vi "hamamatsuReadIndexesOnly.vi"   [LabVIEW 2017]
uses:
  globalDevices.vi
  globalUtilities.vi
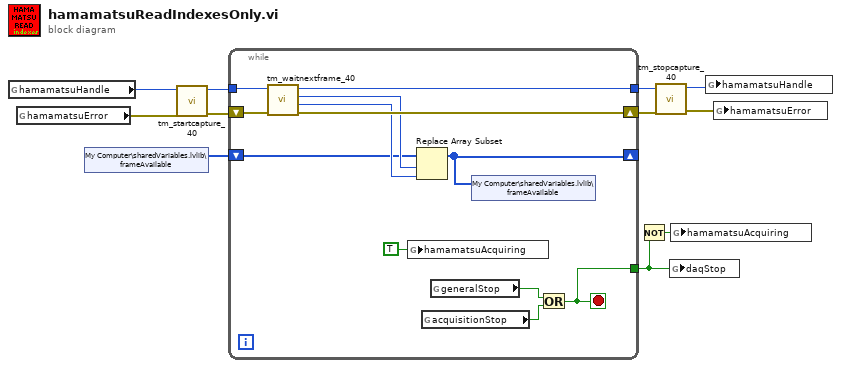
[diagram p0: block diagram]
diagram:
  n1 = global read "globalDevices.vi" "hamamatsuHandle"() -> (w7:u32)
  n2 = global read "globalDevices.vi" "hamamatsuError"() -> (w6:errorcluster)
  n3 = shared-variable "My Computer\\sharedVariables.lvlib\\frameAvailable"() -> (w10:i32[])  [unwired: 1 in, 1 out]
  n4 = call <userlib>:"tm_startcapture_40.vi"("error in (no error)"=w6, "Handle in"=w7) -> ("error out"=w9:errorcluster, "Handle out"=w8:u32)  [unwired: 8 in]
  n5 = while {
    tunnel: w8 -> [w23]
    shift-right: [w19] -> w11
    shift-left: w9 -> [w22]
    shift-right: [w15] -> _
    shift-left: w10 -> [w16]
    tunnel: [w14] -> w5
    tunnel: [w13] -> w2
    stop <- w13 stop-if-true
    n6 = call <userlib>:"tm_waitnextframe_40.vi"("error in (no error)"=w22, "Handle in"=w23) -> ("error out"=w19:errorcluster, "Frame Count"=w17:i32, "Frame Index"=w18:i32, "Handle out"=w14:u32)  [unwired: 6 in]
    n7 = global write "globalUtilities.vi" "hamamatsuAcquiring"(TRUE ("hamamatsuAcquiring")) -> ()
    n8 = Replace Array Subset(array=w16, new element=w17, index=w18) -> (w15:i32[])
    n9 = global read "globalUtilities.vi" "acquisitionStop"() -> (w20:bool)
    n10 = global read "globalUtilities.vi" "generalStop"() -> (w21:bool)
    n11 = shared-variable "My Computer\\sharedVariables.lvlib\\frameAvailable"(w15) -> ()  [unwired: 1 in, 1 out]
    n12 = Or(x=w21, y=w20) -> (x .or. y?=w13:bool)
  }
  n13 = Not(x=w2) -> (.not. x?=w1:bool)
  n14 = call <userlib>:"tm_stopcapture_40.vi"("error in (no error)"=w11, "Handle in"=w5) -> ("error out"=w3:errorcluster, "Handle out"=w4:u32)  [unwired: 8 in]
  n15 = global write "globalUtilities.vi" "daqStop"(w2) -> ()
  n16 = global write "globalUtilities.vi" "hamamatsuAcquiring"(w1) -> ()
  n17 = global write "globalDevices.vi" "hamamatsuHandle"(w4) -> ()
  n18 = global write "globalDevices.vi" "hamamatsuError"(w3) -> ()
